vi "Img Update b Box.vi"(8 "error in (no error)":errorcluster, 11 "LF2R IDE in":refnum<class "Main Panel.lvclass">) -> (0 "error out":errorcluster, 3 "LF2R IDE out":refnum<class "Main Panel.lvclass">)   [LabVIEW 2018, in "Main Panel.lvlib" / "Main Panel.lvclass"]
uses:
  Main Panel.lvclass
  Image/Image Process.lvclass
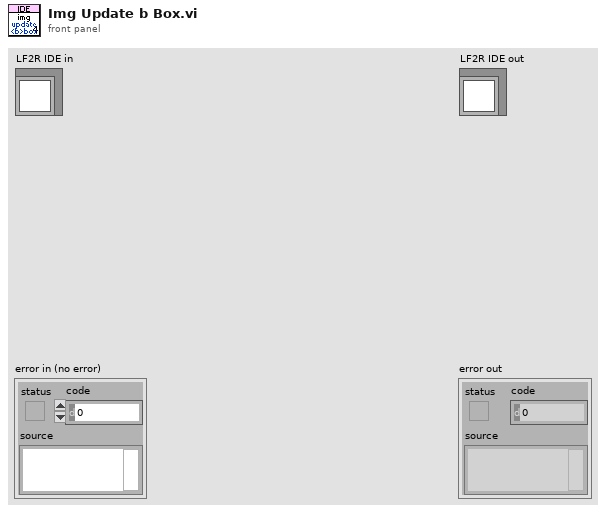
[diagram p1: front panel]
types:
  T1 = typedef "IMAQ Image.ctl" = refnum<image>
  T2 = typedef "Data Parser.lvclass/frame b data.ctl" = cluster{"kind":string, "x":string, "y":string, "w":string, "h":string}
  T3 = cluster{"Fill Color":u32, "Border Color":u32, "Show?":bool}
  T4 = cluster{"x":string, "y":string, "w":string, "h":string}
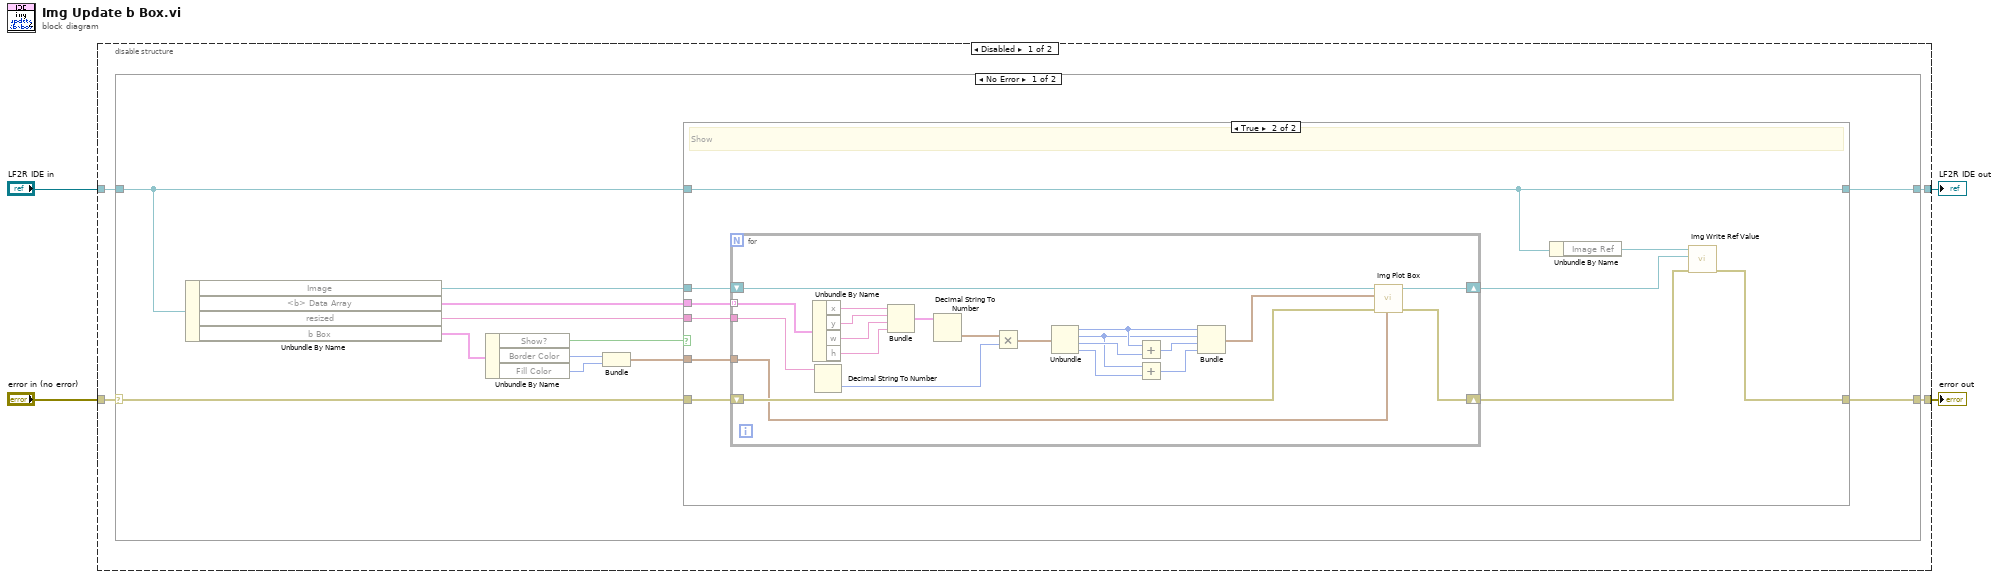
[diagram p0: block diagram]
diagram:
  n1 = disable-structure shown="Disabled" {
    disable-tunnel: "error in (no error)" -> [w8 w57]
    disable-tunnel: [w7 w57] -> w3
    disable-tunnel: "LF2R IDE in" -> [w6 w58]
    disable-tunnel: [w5 w58] -> w1
    frame Disabled {
      n2 = case shown="No Error" w8 {
        selector: w8 -> [w18 w56]
        tunnel: [w16 w56] -> w7
        tunnel: [w12 w55] -> w5
        tunnel: w6 -> [w17 w55]
        frame No Error {
          n3 = Unbundle By Name(w17) -> ("Image"=w20:T1, "<b> Data Array"=w19:T2[], "resized"=w15:string, "b Box"=w14:T3)
          n4 = Unbundle By Name(w14) -> ("Show?"=w13:bool, "Border Color"=w11:u32, "Fill Color"=w10:u32)
          n5 = Bundle("Border Color"=w11, "Fill Color"=w10) -> (w9:cluster{"Border Color":u32, "Fill Color":u32})  [unwired: 1 in]
          n6 = case shown="True" w13 {
            tunnel: w20 -> [_ w32]
            tunnel: w19 -> [_ w31]
            tunnel: w18 -> [w21 w30]
            tunnel: w17 -> [w22 w24]
            tunnel: [w21 w26] -> w16
            tunnel: w15 -> [_ w25]
            tunnel: [w22 w24] -> w12
            tunnel: w9 -> [_ w23]
            frame False {
              # "Skip"
            }
            frame True {
              # "Show"
              n7 = for {
                tunnel: w31 -> [w53] mode=indexing
                shift-right: [w49] -> w27
                shift-left: w30 -> [w50]
                shift-right: [w48] -> w28
                shift-left: w32 -> [w54]
                tunnel: w25 -> [w35]
                tunnel: w23 -> [w33]
                n8 = Unbundle By Name(w53) -> ("x"=w47:string, "y"=w46:string, "w"=w45:string, "h"=w44:string)
                n9 = Decimal String To Number(string=w35) -> (number=w34:i32)  [unwired: 2 in, 1 out]
                n10 = Bundle("x"=w47, "y"=w46, "w"=w45, "h"=w44) -> (w43:T4)  [unwired: 1 in]
                n11 = Decimal String To Number(string=w43) -> (number=w37:cluster{"x":i32, "y":i32, "w":i32, "h":i32})  [unwired: 2 in, 1 out]
                n12 = Multiply(x=w37, y=w34) -> (x*y=w36:cluster{"x":i32, "y":i32, "w":i32, "h":i32})
                n13 = Unbundle(w36) -> ("x"=w42:i32, "y"=w40:i32, "w"=w41:i32, "h"=w39:i32)
                n14 = Add(x=w42, y=w41) -> (x+y=w52:i32)
                n15 = Add(x=w40, y=w39) -> (x+y=w51:i32)
                n16 = Bundle("x"=w42, "y"=w40, w52, w51) -> (w38:cluster{"x":i32, "y":i32, i32, i32})  [unwired: 1 in]
                n17 = call "Img Plot Box.vi"("Color"=w33, "error in (no error)"=w50, "Rectangle"=w38, "Image in"=w54) -> ("error out"=w49:errorcluster, "Image Out"=w48:T1)  [unwired: 6 in]
              }
              n18 = Unbundle By Name(w24) -> ("Image Ref"=w29:refnum<vi>)
              n19 = call "Img Write Ref Value.vi"("error in (no error)"=w27, "Image"=w28, "Image Ref"=w29) -> ("error out"=w26:errorcluster)  [unwired: 8 in]
            }
          }
        }
        frame Error {
        }
      }
    }
    frame Enabled {
    }
  }
  "error out" <- w3
  "LF2R IDE out" <- w1
